vi "Coord window-Add coordinates row.vi"() -> (0 "error out":errorcluster)   [LabVIEW 2013]
uses:
  Globals/Coord window-Globals.vi
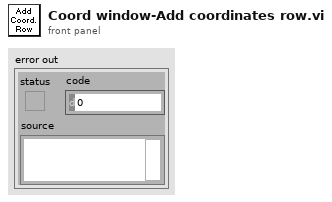
[diagram p1: front panel]
types:
  T1 = typedef "Coordinate list window refs.ctl" = cluster{"Window Name (i.e. Key)":string, "menu reference":refnum<k9>, "VI's reference":refnum<vi>, "Pane 1":refnum<vi>, "Pane 2":refnum<vi>, "Coord Listbox":refnum<vi>, "File name":refnum<vi>, "Picture Map":refnum<vi>, "Stage XYZ Position ind.":refnum<vi>}
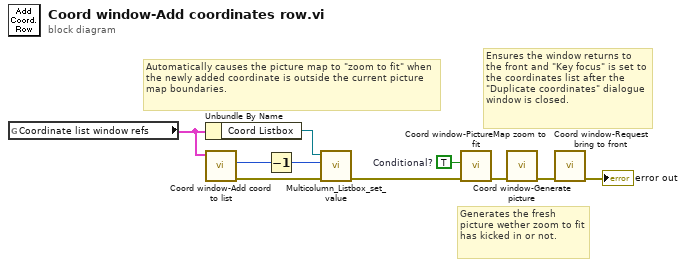
[diagram p0: block diagram]
diagram:
  w3 = TRUE  # Conditional?
  # "Ensures the window returns to the front and \"Key focus\" is set to the coordinates list after the \"Duplicate coordinates\" dialogue window is closed."
  # "Generates the fresh picture wether zoom to fit has kicked in or not."
  # "Automatically causes the picture map to \"zoom to fit\" when the newly added coordinate is outside the current picture map boundaries."
  n1 = global read "Coord window-Globals.vi" "Coordinate list window refs"() -> (w10:T1)
  n2 = Unbundle By Name(w10) -> ("Coord Listbox"=w5:refnum<vi>)
  n3 = call "Coord window-Add coord to list.vi"("Coordinate list window refs"=w10) -> ("error out"=w4:errorcluster, "Number of rows"=w6:i32)  [unwired: 9 in]
  n4 = Decrement(x=w6) -> (x-1=w7:i32)
  n5 = call "Multicolumn_Listbox_set_value.vi"("error in"=w4, "MCListbox value (sel index)"=w7, "Test-Plan Table (in)"=w5) -> ("error out"=w8:errorcluster)  [unwired: 7 in, 1 out]
  n6 = call "Coord window-PictureMap zoom to fit.vi"("error in"=w8, "Conditional?"=w3) -> ("error out"=w9:errorcluster)  [unwired: 9 in]
  n7 = call "Coord window-Generate picture.vi"("error in (no error)"=w9) -> ("error out"=w2:errorcluster)  [unwired: 10 in]
  n8 = call "Coord window-Request bring to front.vi"("error in (no error)"=w2) -> ("error out"=→"error out":errorcluster)  [unwired: 10 in]
